vi "Matrix (2D) to Array (2D).vi"(1 "Matrix":T1=[[3.0, 5.0, 7.0], [4.0, 6.0, 8.0]], 3 "element":dbl format="%#_13g", 5 "Zero Pad":bool) -> (15 "Array":dbl[][](array[numeric])=[[3.0, 5.0, 7.0], [4.0, 6.0, 8.0]])   [LabVIEW 2014]
uses:
  <vilib>/Analysis/Matrix/Datatypes/RealMatrix.ctl
  <vilib>/Analysis/Matrix/NI_Matrix.lvlib
panel:
  out "#rows":i32=2
  out "#cols":i32=3
  out "#rows":i32=2
  out "#cols":i32=3
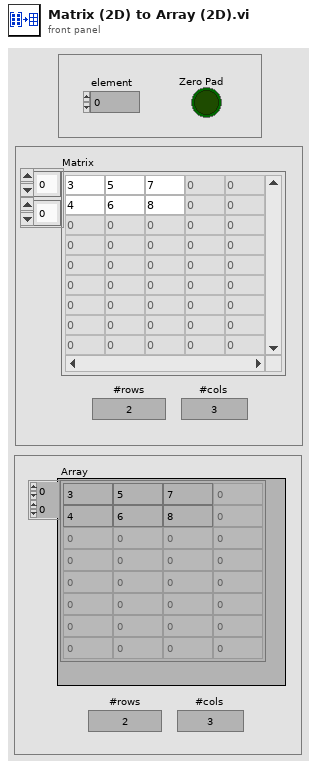
[diagram p1: front panel]
types:
  T1 = typedef "NI_Matrix.lvlib/RealMatrix.ctl" = dbl[][]
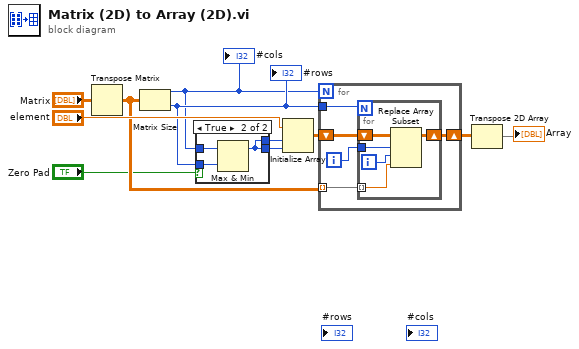
[diagram p0: block diagram]
diagram:
  n1 = Transpose Matrix(1:"Matrix") -> (0:w8:T1)
  n2 = Matrix Size(0:w8) -> (1:w3:i32, 2:w4:i32)
  "#cols" <- w3
  "#rows" <- w4
  n3 = case shown="True" "Zero Pad" {
    tunnel: w4 -> [w12 w15]
    tunnel: w3 -> [w13 w16]
    tunnel: [w13 w14] -> w1
    tunnel: [w12 w14] -> w2
    frame False {
    }
    frame True {
      n4 = Max & Min(x=w16, y=w15) -> (max(x,y)=w14:i32)  [unwired: 1 out]
    }
  }
  n5 = Initialize Array("element", w1, w2) -> (w9:dbl[][])
  n6 = for {
    N: w3 -> [_]
    tunnel: w4 -> [w21]
    shift-right: [w19] -> w6
    shift-left: w9 -> [w20]
    tunnel: w8 -> [w17] mode=indexing
    i -> [w18]
    n7 = for {
      N: w21 -> [_]
      shift-right: [w25] -> w19
      shift-left: w20 -> [w26]
      tunnel: w18 -> [w24]
      tunnel: w17 -> [w22] mode=indexing
      i -> [w23]
      n8 = Replace Array Subset(array=w26, new element=w22, index (row)=w24, index (col)=w23) -> (w25:dbl[][])
    }
  }
  n9 = Transpose 2D Array(2D array=w6) -> (transposed array=→"Array":dbl[][])
